vi "Convert IMAQ Image to Picture.vi"(11 "Image In":T1) -> (3 "new picture":picture)   [LabVIEW 2020]
uses:
  <vilib>/vision/Image Controls.llb/IMAQ Image.ctl
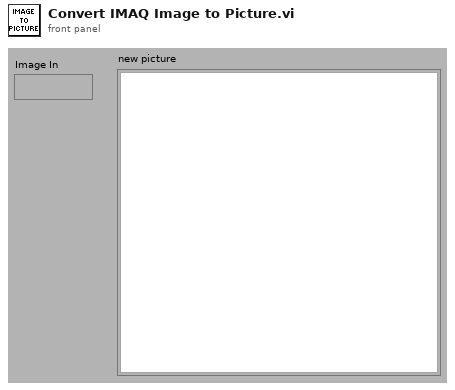
[diagram p1: front panel]
types:
  T1 = typedef "IMAQ Image.ctl" = refnum<image>
  T2 = typedef "imagedata.ctl" = cluster{"image type":i32, "image depth":i32, "image":u8[], "mask":u8[], "colors":u32[], "Rectangle":cluster{"left":i16, "top":i16, "right":i16, "bottom":i16}}
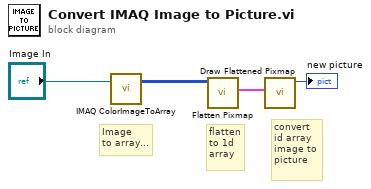
[diagram p0: block diagram]
diagram:
  # "convert\nid array\nimage to\npicture"
  # "flatten\nto 1d \narray"
  # "Image\nto array..."
  n1 = call "IMAQ ColorImageToArray"("Image"="Image In") -> ("Image Pixels (U32)"=w1:u32[][])  [unwired: 3 in, 2 out]
  n2 = call <vilib>:"Flatten Pixmap.vi"("24-bit pixmap"=w1) -> ("image data"=w3:T2)  [unwired: 5 in, 5 out]
  n3 = call <vilib>:"Draw Flattened Pixmap.vi"("image data"=w3) -> ("new picture"=→"new picture":picture)  [unwired: 1 in, 7 out]
